vi "GetSpData.vi"(0 "VISA resource name":refnum<visa-resource-name>, 5 "S11 file path":path=path "C:/RageATE/Instruments/Agilent N5232A PNA-L/Labview Driver/RageATE-PNA/S11_1.tmp", 11 "error in (no error)":errorcluster, 12 "F(Units)":i32(ring) items=["Hz", "KHz", "MHz", "GHz"]) -> (3 "Freq(ary)":dbl[](array[numeric]), 4 "VISA resource name out":refnum<visa-resource-name>, 15 "error out":errorcluster)   [LabVIEW 2018]
doc: "Sets the start frequency and stop frequency of the analyzer."
uses:
  <vilib>/Utility/file.llb/Write Delimited Spreadsheet (DBL).vi
  Initialize References/Sequence Globals.vi
  Keysight PNA Series/Keysight PNA Series.lvlib
panel:
  out "Numeric":i32
  out "Array":bool[](array[boolean])
  out "S11_Temp":path
  out "AVG?(t)":bool
  out "Error Message":string
  out "AvgMode?":string
  out "AvgState?":string
  out "AvgCount?(str)":string
  in  "CHANNEL":i32=1
  out "SWE-MODE?":string
  out "Avg Count?(num)":i32
  out "Sweep Complete(?)b":bool
  out "Trace":dbl[][](array[numeric])
  out "Data":dbl[](array[numeric])
  out "NumPoi":dbl
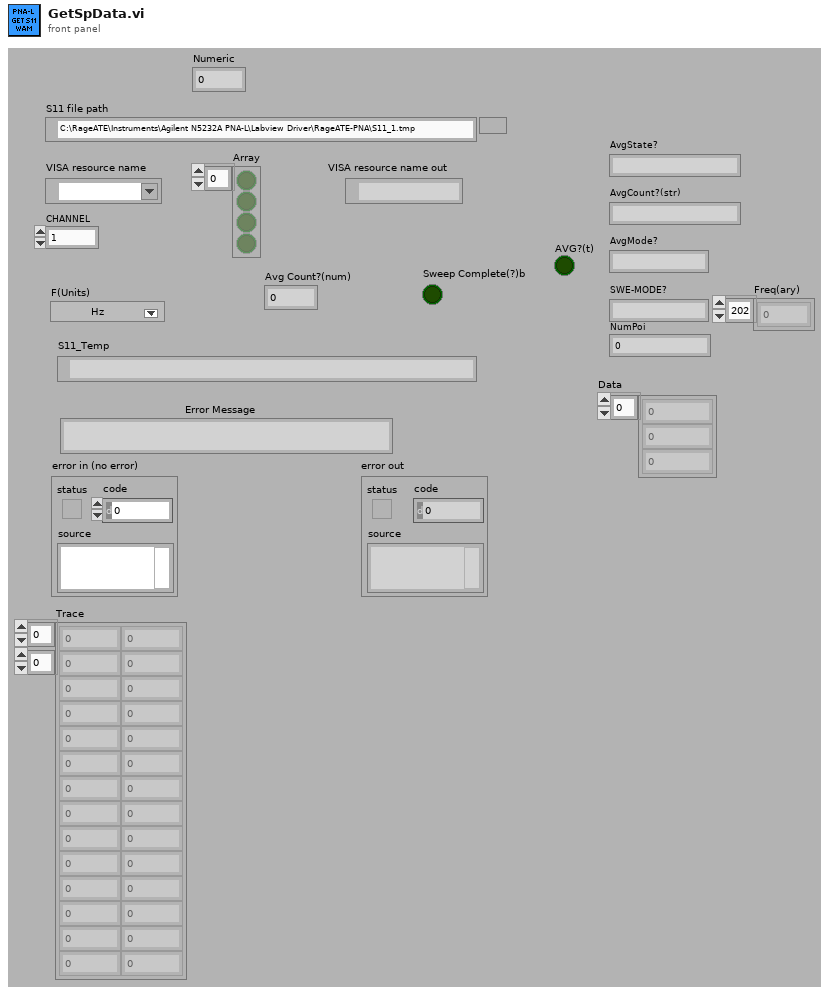
[diagram p1: front panel]
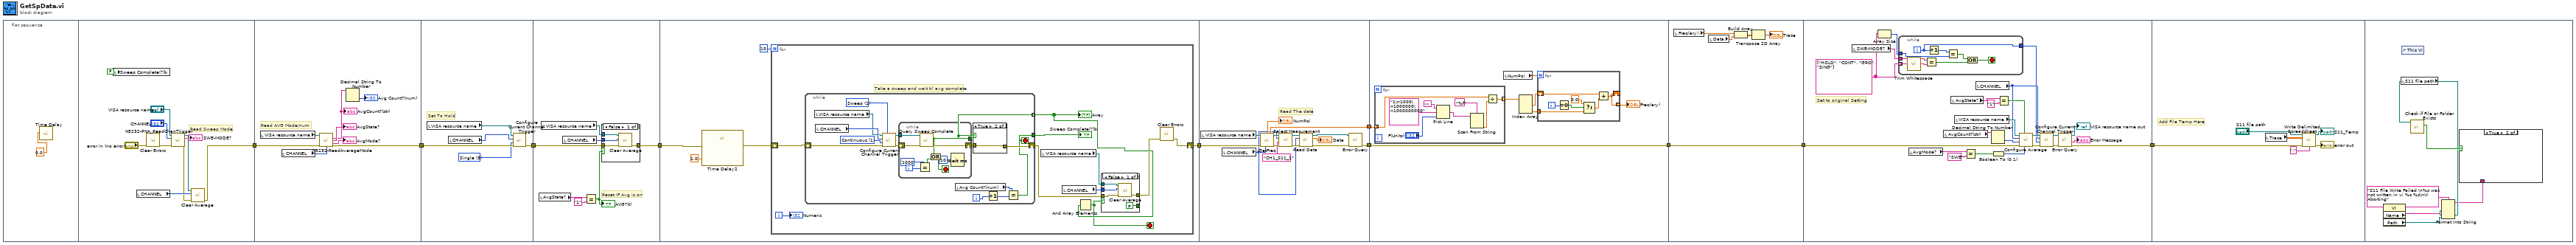
[diagram p0: block diagram]
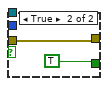
[diagram p3: hidden frame]
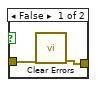
[diagram p4: hidden frame]
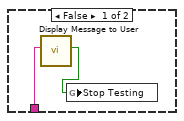
[diagram p5: hidden frame]
diagram:
  n1 = flat-sequence {
    tunnel: [w12] -> w9
    tunnel: w9 -> [w28]
    tunnel: [w24] -> w8
    tunnel: w8 -> [w33]
    tunnel: [w34] -> w7
    tunnel: w7 -> [w38]
    tunnel: [w35] -> w6
    tunnel: w6 -> [w50]
    tunnel: [w51] -> w4
    tunnel: [w108] -> w10
    tunnel: w4 -> [w102]
    tunnel: [w101] -> w1
    tunnel: w10 -> [w115]
    tunnel: [w109] -> w2
    tunnel: w1 -> [w109]
    tunnel: [w132] -> w3
    tunnel: w2 -> [w132]
    tunnel: [w158] -> w5
    tunnel: w3 -> [w157]
    tunnel: w5 -> [w172]
    frame #0 {
      n2 = call "Time Delay"("Delay Time (s)"=0.0) -> ()  [unwired: 10 in, 1 out]
    }
    frame #1 {
      # "Read Sweep Mode"
      n3 = local write "Sweep Complete(?)b"(FALSE ("Sweep Complete")) -> ()
      n4 = local read "CHANNEL"() -> (w14:i32)
      n5 = call <vilib>:"Clear Errors.vi"("error in (no error)"="error in (no error)") -> ("error out"=w17:errorcluster)  [unwired: 5 in, 1 out]
      n6 = call "N5232-PNA_ReadChanTrigger.vi"("Session In"="VISA resource name", "CHANNEL"="CHANNEL", "error in"=w17) -> ("Session Out"=w15:refnum<visa-resource-name>, "SWE-MODE?"=→"SWE-MODE?":string, "error out"=w13:errorcluster)  [unwired: 8 in, 2 out]
      n7 = call "Clear Average.vi"("error in (no error)"=w13, "Channel (1)"=w14, "VISA resource name"=w15) -> ("error out"=w12:errorcluster)  [unwired: 7 in, 1 out]
    }
    frame #2 {
      # "Read AVG Mode/num"
      n8 = local read "VISA resource name"() -> (w29:refnum<visa-resource-name>)
      n9 = local read "CHANNEL"() -> (w27:i32)
      n10 = call "N5232-ReadAverageMode.vi"("Session In"=w29, "error in"=w28, "Chan"=w27) -> ("AvgCount?"=w23:string, "AvgState?"=→"AvgState?":string, "AvgMode?"=→"AvgMode?":string, "error out"=w24:errorcluster)  [unwired: 8 in, 1 out]
      "AvgCount?(str)" <- w23
      n11 = Decimal String To Number(string=w23) -> (number=→"Avg Count?(num)":i32)  [unwired: 2 in, 1 out]
    }
    frame #3 {
      w32 = 3 items=["Hold", "Continuous", "Groups", "Single"] ("Trigger Condition (1: Continuous)")
      # "Set To Hold"
      n12 = local read "VISA resource name"() -> (w31:refnum<visa-resource-name>)
      n13 = local read "CHANNEL"() -> (w30:i32)
      n14 = call "Configure Current Channel Trigger.vi"("error in (no error)"=w33, "Trigger Condition (1: Continuous)"=w32, "Channel (1)"=w30, "VISA resource name"=w31) -> ("error out"=w34:errorcluster)  [unwired: 6 in, 1 out]
    }
    frame #4 {
      # "Reset IF Avg is on"
      n15 = local read "AvgState?"() -> (w41:string)
      n16 = local read "VISA resource name"() -> (w37:refnum<visa-resource-name>)
      n17 = local read "CHANNEL"() -> (w36:i32)
      n18 = Equal?(x=w41, y="1") -> (x = y?=w39:bool)
      "AVG?(t)" <- w39
      n19 = case shown="False" w39 {
        tunnel: w38 -> [w45 w46]
        tunnel: w37 -> [w44 _]
        tunnel: w36 -> [w43 _]
        tunnel: [w42 w46] -> w35
        frame False {
          n20 = call "Clear Average.vi"("error in (no error)"=w45, "Channel (1)"=w43, "VISA resource name"=w44) -> ("error out"=w42:errorcluster)  [unwired: 7 in, 1 out]
        }
        frame True {
        }
      }
    }
    frame #5 {
      n21 = call "Time Delay2"("error in (no error)"=w50, "Delay Time (s)"=1.0) -> ("error out"=w49:errorcluster)  [unwired: 9 in]
      n22 = for {
        N: 10 -> [_]
        shift-right: [w52] -> w51
        shift-left: w49 -> [w61]
        i -> [w60]
        stop <- w54 stop-if-true
        # "Take a sweep and wait til avg complete"
        n23 = while {
          shift-right: [w74] -> w57
          shift-left: w61 -> [w81]
          tunnel: [w71] -> w56
          tunnel: [w69] -> w55 mode=indexing
          i -> [w79]
          stop <- w71 stop-if-true
          w70 = 1 items=["Channel", "Sweep", "Point", "Trace"] ("Trigger Mode (0: Channel)")
          w82 = 1 items=["Hold", "Continuous", "Groups", "Single"] ("Trigger Condition (1: Continuous)")
          n24 = local read "VISA resource name"() -> (w76:refnum<visa-resource-name>)
          n25 = local read "CHANNEL"() -> (w80:i32)
          n26 = call "Configure Current Channel Trigger.vi"("Trigger Mode (0: Channel)"=w70, "error in (no error)"=w81, "Trigger Condition (1: Continuous)"=w82, "Channel (1)"=w80, "VISA resource name"=w76) -> ("error out"=w72:errorcluster, "VISA resource name out"=w73:refnum<visa-resource-name>)  [unwired: 5 in]
          n27 = while {
            tunnel: w73 -> [w90]
            shift-right: [w91] -> w75
            shift-left: w72 -> [w89]
            tunnel: [w88] -> w69
            i -> [w86]
            stop <- w87 stop-if-true
            n28 = Equal?(x=1000, y=w86) -> (x = y?=w85:bool)
            n29 = call "Query Sweep Complete.vi"("error in (no error)"=w89, "VISA resource name"=w90) -> ("error out"=w91:errorcluster, "Sweep Complete"=w88:bool)  [unwired: 7 in, 1 out]
            n30 = Or(x=w88, y=w85) -> (x .or. y?=w87:bool)
            n31 = Wait (ms)(milliseconds to wait=u32 10) -> ()  [unwired: 1 out]
          }
          n32 = local read "Avg Count?(num)"() -> (w77:i32)
          n33 = case shown="True" w69 {
            tunnel: w75 -> [w93 w94]
            tunnel: [w92 w94] -> w74
            frame False {
              n34 = call <vilib>:"Clear Errors.vi"("error in (no error)"=w93) -> ("error out"=w92:errorcluster)  [unwired: 5 in, 1 out]
            }
            frame True {
            }
          }
          n35 = Increment(x=w79) -> (x+1=w78:i32)
          n36 = Equal?(x=w77, y=w78) -> (x = y?=w71:bool)
        }
        "Sweep Complete(?)b" <- w56
        "Array" <- w55
        n37 = local read "VISA resource name"() -> (w59:refnum<visa-resource-name>)
        n38 = local read "CHANNEL"() -> (w58:i32)
        n39 = And Array Elements(Boolean array=w55) -> (logical AND=w54:bool)
        n40 = case shown="False" w54 {
          tunnel: w59 -> [w66 _]
          tunnel: w58 -> [w65 _]
          tunnel: [w64 w68] -> w53
          tunnel: w57 -> [w63 w68]
          tunnel: [FALSE TRUE] -> _
          frame False {
            n41 = call "Clear Average.vi"("error in (no error)"=w63, "Channel (1)"=w65, "VISA resource name"=w66) -> ("error out"=w64:errorcluster)  [unwired: 7 in, 1 out]
          }
          frame True {
          }
        }
        n42 = call <vilib>:"Clear Errors.vi"("error in (no error)"=w53) -> ("error out"=w52:errorcluster)  [unwired: 5 in, 1 out]
        "Numeric" <- w60
      }
    }
    frame #6 {
      # "Read The data"
      n43 = local read "VISA resource name"() -> (w103:refnum<visa-resource-name>)
      n44 = local read "CHANNEL"() -> (w95:i32)
      n45 = call "GetFreq.vi"("Session In"=w103, "error in"=w102, "CHAN(1)"=w95) -> ("NumPoi"=→"NumPoi":dbl, "Freq(ary)"=w108:dbl[], "Session Out"=w99:refnum<visa-resource-name>, "error out"=w96:errorcluster)  [unwired: 9 in]
      n46 = call "Select Measurement.vi"("error in (no error)"=w96, "Measurement Name (CH1_S11_1)"="CH1_S11_1", "Channel (1)"=w95, "VISA resource name"=w99) -> ("error out"=w97:errorcluster, "VISA resource name out"=w100:refnum<visa-resource-name>)  [unwired: 6 in]
      n47 = call "Read Data.vi"("error in (no error)"=w97, "Channel (1)"=w95, "VISA resource name"=w100) -> ("error out"=w105:errorcluster, "Data"=→"Data":dbl[], "VISA resource name out"=w106:refnum<visa-resource-name>)  [unwired: 6 in]
      n48 = call "Error Query.vi"("error in (no error)"=w105, "VISA resource name"=w106) -> ("error out"=w101:errorcluster)  [unwired: 6 in, 3 out]
    }
    frame #7 {
      n49 = for {
        tunnel: w115 -> [w125] mode=indexing
        tunnel: [w123] -> w114 mode=indexing
        n50 = Pick Line(string ("")="", multi-line string="1\n1000\n1000000\n1000000000", line index="F(Units)") -> (output string=w128:string)
        n51 = Scan From String(format string="%f", input string=w128) -> (output 1=w124:dbl)  [unwired: 3 in, 3 out]
        n52 = Divide(x=w125, y=w124) -> (x/y=w123:dbl)
      }
      n53 = local read "NumPoi"() -> (w113:dbl)
      n54 = Index Array(array=w114) -> (element #1=w110:dbl, element #3=w112:dbl)  [unwired: 3 in, 1 out]
      n55 = for {
        N: w113 -> [_]
        tunnel: w112 -> [w117]
        shift-right: [w121] -> _
        shift-left: w110 -> [w122]
        tunnel: [w121] -> w111 mode=indexing
        i -> [w120]
        n56 = Equal To 0?(x=w120) -> (x = 0?=w119:bool)
        n57 = Select(t=0.0 ("f"), s=w119, f=w117) -> (s? t:f=w116:dbl)
        n58 = Add(x=w122, y=w116) -> (x+y=w121:dbl)
      }
      "Freq(ary)" <- w111
    }
    frame #8 {
      n59 = local read "Freq(ary)"() -> (w135:dbl[])
      n60 = local read "Data"() -> (w131:dbl[])
      n61 = Build Array(w135, w131) -> (w134:dbl[][])
      n62 = Transpose 2D Array(2D array=w134) -> (transposed array=→"Trace":dbl[][])
    }
    frame #9 {
      w145 = string[] ["HOLD", "CONT", "GRO", "SING"]
      # "Set to original Setting"
      n63 = local read "SWE-MODE?"() -> (w144:string)
      n64 = Array Size(array=w145) -> (size(s)=w143:i32)
      n65 = while {
        tunnel: w145 -> [w166] mode=indexing
        tunnel: [w161] -> w142
        tunnel: w144 -> [w165]
        tunnel: w143 -> [w162]
        i -> [w161]
        stop <- w163 stop-if-true
        n66 = call <vilib>:"Trim Whitespace.vi"("string"=w166) -> ("trimmed string"=w164:string)  [unwired: 1 in]
        n67 = Equal?(x=w165, y=w164) -> (x = y?=w167:bool)
        n68 = Increment(x=w161) -> (x+1=w160:i32)
        n69 = Equal?(x=w160, y=w162) -> (x = y?=w159:bool)
        n70 = Or(x=w159, y=w167) -> (x .or. y?=w163:bool)
      }
      n71 = local read "AvgMode?"() -> (w154:string)
      n72 = local read "AvgCount?(str)"() -> (w155:string)
      n73 = local read "AvgState?"() -> (w150:string)
      n74 = local read "VISA resource name"() -> (w156:refnum<visa-resource-name>)
      n75 = Equal?(x=w154, y="SWE") -> (x = y?=w152:bool)
      n76 = local read "CHANNEL"() -> (w136:i32)
      n77 = Decimal String To Number(string=w155) -> (number=w141:i32)  [unwired: 2 in, 1 out]
      n78 = Boolean To (0,1)(Boolean=w152) -> (0, 1=w151:i16)
      n79 = Equal?(x=w150, y="1") -> (x = y?=w148:bool)
      n80 = call "Configure Average.vi"("Average Mode (1: Sweep)"=w151, "Enable Average (F: Disable)"=w148, "error in (no error)"=w157, "Average Count (1)"=w141, "Channel (1)"=w136, "VISA resource name"=w156) -> ("error out"=w146:errorcluster, "VISA resource name out"=w147:refnum<visa-resource-name>)  [unwired: 4 in]
      n81 = call "Configure Current Channel Trigger.vi"("error in (no error)"=w146, "Trigger Condition (1: Continuous)"=w142, "Channel (1)"=w136, "VISA resource name"=w147) -> ("error out"=w140:errorcluster, "VISA resource name out"=w139:refnum<visa-resource-name>)  [unwired: 6 in]
      n82 = call "Error Query.vi"("error in (no error)"=w140, "VISA resource name"=w139) -> ("error out"=w158:errorcluster, "Error Message"=→"Error Message":string, "VISA resource name out"=→"VISA resource name out":refnum<visa-resource-name>)  [unwired: 6 in, 1 out]
    }
    frame #10 {
      # "Add File Temp Here"
      n83 = local read "Trace"() -> (w171:dbl[][])
      n84 = call-poly <vilib>:"Write Delimited Spreadsheet.vi"("file path (dialog if empty)"="S11 file path", "2D data"=w171, "error in (no error)"=w172, "delimiter (\\t)"="," ("delimiter (\\t)")) -> ("new file path (Not A Path if cancelled)"=→"S11_Temp":path, "error out"=→"error out":errorcluster)  [unwired: 10 in]
    }
    frame #11 {
      w176 = "S11 File Write Failed \n%s was not written in vi %s %s\nVi Aborting" ("format string")
      n85 = property class="VI" props=["Name", "Path"]() -> ("Path"=w175:path)  [unwired: 2 in, 3 out]
      n86 = local read "S11 file path"() -> (w177:path)
      n87 = control-ref of="This VI"() -> ()  [unwired: 1 out]
      n88 = call <vilib>:"Check if File or Folder Exists.vi"("path"=w177) -> ("file or folder exists?"=w178:bool)  [unwired: 8 in, 2 out]
      n89 = Format Into String(format string=w176, w177, w176, w175) -> (resulting string=w174:string)  [unwired: 2 in, 1 out]
      n90 = case shown="True" w178 {
        tunnel: w174 -> [w180 _]
        frame False {
          n91 = call "Display Message to User"("Message"=w180) -> ("OK"=w179:bool)  [unwired: 9 in, 1 out]
          n92 = global write "Sequence Globals.vi" "Stop Testing"(w179) -> ()
        }
        frame True {
        }
      }
    }
  }
